vi "update channels to match type definitions.vi"(8 "error in":errorcluster, 11 "fixed channel configuration in":refnum<class "fixed channel configuration.lvclass">) -> (0 "error out":errorcluster, 3 "fixed channel configuration out":refnum<class "fixed channel configuration.lvclass">)   [LabVIEW 2013, in "fixed channel configuration.lvclass"]
uses:
  fixed channel configuration.lvclass
  fixed channel configuration.lvclass/fixed channel configuration.ctl
  <vilib>/NI/Tag Bus/tag/tag descriptor.lvclass/tag descriptor.ctl
  <vilib>/NI/Tag Bus Module Framework/channel/TBM channel.lvclass/TBM channel.ctl
  <vilib>/NI/Tag Bus/tag/read data type.vi
  <vilib>/NI/Tag Bus Module Framework/channel/Read channel classification.vi
  <vilib>/NI/Tag Bus/tag/read tag name.vi
  <vilib>/NI/Tag Bus/tag/tag descriptor.lvclass
  <vilib>/NI/Tag Bus Module Framework/channel/TBM channel.lvclass
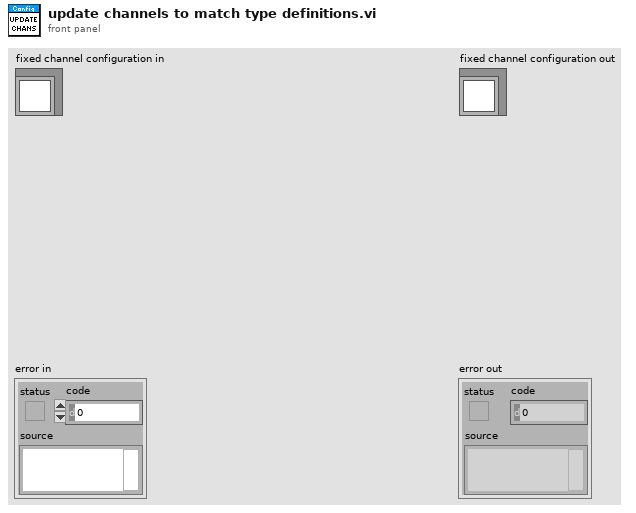
[diagram p1: front panel]
types:
  T1 = typedef "tag bus.lvlib/tag descriptor.lvclass/Data Type.ctl" = enum16{"Double", "Single", "I64", "I32", "I16", "I8", "U64", "U32", "U16", "U8", "Boolean", "String", "Array of Double", "Array of Single", "Array of I64", "Array of I32", "Array of I16", "Array of I8", "Array of U64", "Array of U32", "Array of U16", "Array of U8", "Array of Boolean", "Array of String"}
  T2 = typedef "TBM channel.lvclass/channel classification.ctl" = enum16{"input data", "output data", "processing parameter", "processing result"}
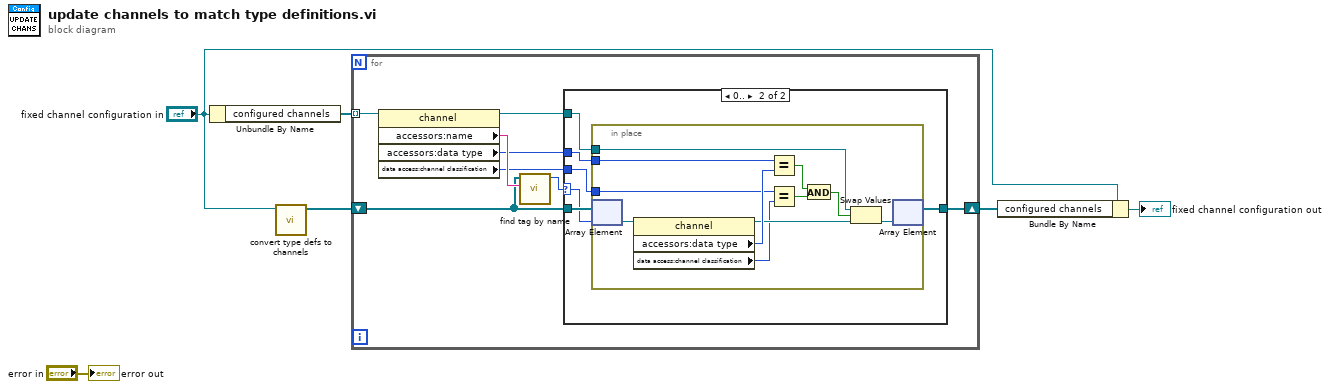
[diagram p0: block diagram]
diagram:
  n1 = Unbundle By Name("fixed channel configuration in") -> ("configured channels"=w4:refnum<class "TBM channel.lvclass">[])
  n2 = call "convert type defs to channels.vi"("fixed channel configuration"="fixed channel configuration in") -> ("Array out"=w6:refnum<class "TBM channel.lvclass">[])  [unwired: 9 in, 1 out]
  n3 = for {
    shift-right: [w10] -> w5
    shift-left: w6 -> [w11]
    tunnel: w4 -> [w14] mode=indexing
    n4 = property class="channel"(reference=w14) -> (reference out=w8:refnum<class "TBM channel.lvclass">, "accessors:name"=w13:string, "accessors:data type"=w9:T1, "data access:channel classification"=w7:T2)  [unwired: 1 in, 1 out]
    n5 = call <vilib>:"find tag by name.vi"("name"=w13, "tags in"=w11) -> ("index"=w12:i32)  [unwired: 9 in]
    n6 = case shown="0.." w12 {
      selector: w12 -> [_ w20]
      tunnel: w11 -> [w15 w21]
      tunnel: [w15 w19] -> w10
      tunnel: w9 -> [_ w18]
      tunnel: w8 -> [_ w17]
      tunnel: w7 -> [_ w16]
      frame ..-1 {
      }
      frame 0.. {
        n7 = in-place {
          in-place-border: w18 -> [w30]
          in-place-border: w17 -> [w27]
          in-place-border: w16 -> [w23]
          n8 = in-place-array #1(w21, w20) -> (w32:refnum<class "TBM channel.lvclass">)
          n9 = property class="channel"(reference=w32) -> (reference out=w29:refnum<class "TBM channel.lvclass">, "accessors:data type"=w31:T1, "data access:channel classification"=w24:T2)  [unwired: 1 in, 1 out]
          n10 = Equal?(x=w30, y=w31) -> (x = y?=w26:bool)
          n11 = Equal?(x=w23, y=w24) -> (x = y?=w22:bool)
          n12 = And(x=w26, y=w22) -> (x .and. y?=w25:bool)
          n13 = Swap Values(12:w27, 13:w25, 14:w29) -> (3:w28:refnum<class "TBM channel.lvclass">)  [unwired: 1 out]
          n14 = in-place-array #1(w28) -> (w19:refnum<class "TBM channel.lvclass">[])  [unwired: 1 out]
        }
      }
    }
  }
  n15 = Bundle By Name(cluster="fixed channel configuration in", "configured channels"=w5) -> (→"fixed channel configuration out":refnum<class "fixed channel configuration.lvclass">)
  "error out" <- "error in"
